vi "To Double.vi"(8 "error in (no error)":errorcluster, 11 "SensorData in":refnum<class "SensorData.lvclass">) -> (0 "error out":errorcluster, 2 "Value":dbl, 3 "SensorData out":refnum<class "SensorData.lvclass">)   [LabVIEW 2012, in "Sensor Definition.lvlib" / "SensorData.lvclass"]
uses:
  SensorData.lvclass
  <vilib>/Utility/error.llb/Error Cluster From Error Code.vi
  <vilib>/ErrorRing/Error Ring.xnode
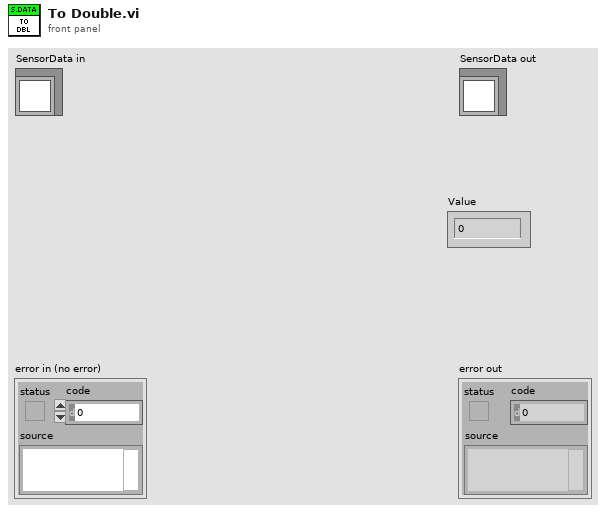
[diagram p1: front panel]
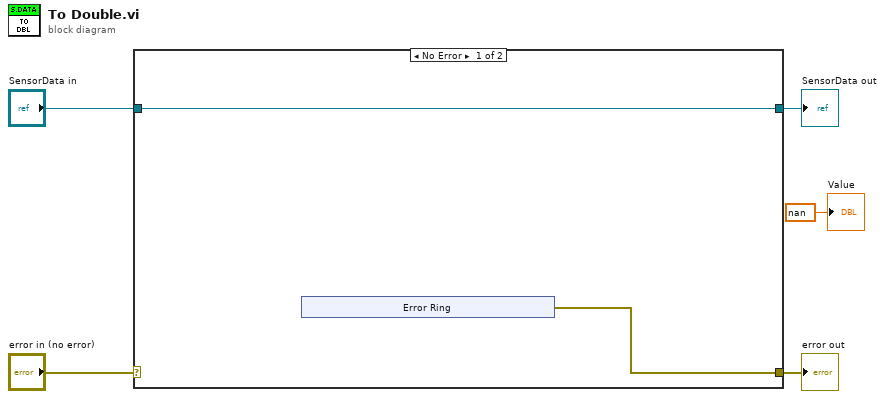
[diagram p0: block diagram]
diagram:
  n1 = case shown="No Error" "error in (no error)" {
    selector: "error in (no error)" -> [_ w14]
    tunnel: [w6 w14] -> w4
    tunnel: [w7 w13] -> w2
    tunnel: "SensorData in" -> [w7 w13]
    frame No Error {
      n2 = xnode "Error Ring"() -> ("error out"=w6:errorcluster)
    }
    frame Error {
    }
  }
  "error out" <- w4
  "SensorData out" <- w2
  "Value" <- nan ("Value")
